vi "Fetch Multi Eval Meas List Segment Total TX Power Results.vi"(6 "Segment (1)":T2=1, 8 "error in (no error)":errorcluster, 9 "Result Type (Current)":i32(ring) items=["Current"=0, "Average"=1, "Standard Deviation"=3, "Maximum"=4, "Minimum"=5], 10 "Instance (1)":T3=1, 11 "VISA resource name":refnum<visa-resource-name>) -> (0 "error out":errorcluster, 1 "TX Power":dbl format="%^.3e", 2 "Reliability":T1, 3 "VISA resource name out":refnum<visa-resource-name>, 4 "Expired Statistics":i32, 5 "Out Of Tolerance":i32)   [LabVIEW 2020, in "Rohde&Schwarz CMWXP NR FR1 Measurement.lvlib"]
doc: "Return total TX power results for segment <no> in list mode.\n\nAttributes:\nRSCMWXPNRFR1M_ATTR_FETCH_MULTI_EVAL_MEAS_LIST_SEGMENT_TOTAL_TX_POWER_CURRENT_RESULTS\nRSCMWXPNRFR1M_ATTR_FETCH_MULTI_EVAL_MEAS_LIST_SEGMENT_TOTAL_TX_POWER_AVERAGE_RESULTS\nRSCMWXPNRFR1M_ATTR_FETCH_MULTI_EVAL_MEAS_LIST_SEGMENT_TOTAL_TX_POWER_STANDARD_DEVIATION_RESULTS\nRSCMWXPNRFR1M_ATTR_FETCH_MULTI_EVAL_MEAS_LIST_SEGMENT_TOTAL_TX_POWER_MAXIMUM_RESULTS\nRSCMWXPNRFR1M_ATTR_FETCH_MULTI_EVAL_MEAS_LIST_SEGMENT_TOTAL_TX_POWER_MINIMUM_RESULTS\n\nRemote-control commands:\nFETCh:NRSub:MEAS<i>:MEValuation:LIST:SEGMent<no>:POWer:CURRent?\nFETCh:NRSub:MEAS<i>:MEValuation:LIST:SEGMent<no>:POWer:AVERage?\nFETCh:NRSub:MEAS<i>:MEValuation:LIST:SEGMent<no>:POWer:SDEViation?\nFETCh:NRSub:MEAS<i>:MEValuation:LIST:SEGMent<no>:POWer:MAXimum?\nFETCh:NRSub:MEAS<i>:MEValuation:LIST:SEGMent<no>:POWer:MINimum?"
uses:
  <instrlib>/Rohde&Schwarz CMWXP NR FR1 Measurement/Rohde&Schwarz CMWXP NR FR1 Measurement.lvlib
  <instrlib>/Rohde&Schwarz CMWXP NR FR1 Measurement/Private/_Instance.ctl
  <instrlib>/Rohde&Schwarz CMWXP NR FR1 Measurement/Private/_Segment.ctl
  <instrlib>/Rohde&Schwarz CMWXP NR FR1 Measurement/Private/_SegReliability.ctl
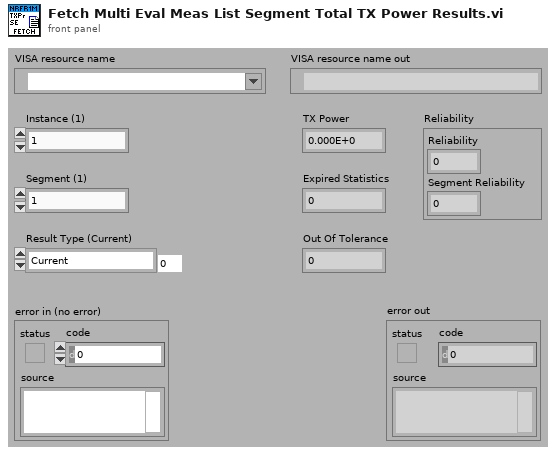
[diagram p1: front panel]
types:
  T1 = typedef "Rohde&Schwarz CMWXP NR FR1 Measurement.lvlib/_SegReliability.ctl" = cluster{"Reliability":i32, "Segment Reliability":i32}
  T2 = typedef "Rohde&Schwarz CMWXP NR FR1 Measurement.lvlib/_Segment.ctl" = i32
  T3 = typedef "Rohde&Schwarz CMWXP NR FR1 Measurement.lvlib/_Instance.ctl" = i32
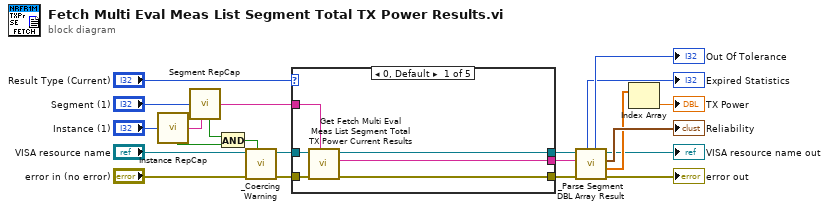
[diagram p0: block diagram]
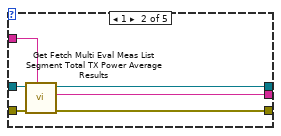
[diagram p2: hidden frame]
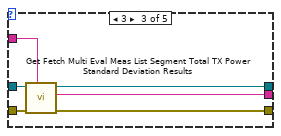
[diagram p3: hidden frame]
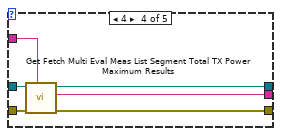
[diagram p4: hidden frame]
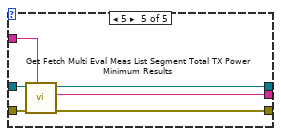
[diagram p5: hidden frame]
diagram:
  n1 = call <instrlib>:"Instance RepCap.vi"("Instance In"="Instance (1)") -> ("In Range?"=w17:bool, "RepCap Identifier Out"=w16:string)  [unwired: 1 in]
  n2 = call <instrlib>:"Segment RepCap.vi"("Segment In"="Segment (1)", "RepCap String In (\"\")"=w16) -> ("In Range?"=w15:bool, "RepCap Identifier Out"=w14:string)
  n3 = And(x=w15, y=w17) -> (x .and. y?=w18:bool)
  n4 = call <instrlib>:"_Coercing Warning.vi"("In Range?"=w18, "error in (no error)"="error in (no error)", "VISA resource name"="VISA resource name") -> ("error out"=w12:errorcluster, "VISA resource name out"=w13:refnum<visa-resource-name>)  [unwired: 7 in]
  n5 = case shown="0, Default" "Result Type (Current)" {
    tunnel: w14 -> [w28 w34 w40 w46 w52]
    tunnel: w13 -> [w27 w33 w39 w45 w51]
    tunnel: w12 -> [w26 w32 w38 w44 w50]
    tunnel: [w25 w31 w37 w43 w49] -> w11
    tunnel: [w24 w30 w36 w42 w48] -> w10
    tunnel: [w23 w29 w35 w41 w47] -> w9
    frame 0, Default {
      n6 = call "Get Fetch Multi Eval Meas List Segment Total TX Power Current Results"("Repeated Capabilities"=w28, "error in (no error)"=w26, "instrument handle"=w27) -> ("error out"=w23:errorcluster, "Fetch Multi Eval Meas List Segment Total TX Power Current Results"=w24:string, "instrument handle out"=w25:refnum<visa-resource-name>)  [unwired: 6 in]
    }
    frame 1 {
      n7 = call "Get Fetch Multi Eval Meas List Segment Total TX Power Average Results"("Repeated Capabilities"=w34, "error in (no error)"=w32, "instrument handle"=w33) -> ("error out"=w29:errorcluster, "Fetch Multi Eval Meas List Segment Total TX Power Average Results"=w30:string, "instrument handle out"=w31:refnum<visa-resource-name>)  [unwired: 6 in]
    }
    frame 3 {
      n8 = call "Get Fetch Multi Eval Meas List Segment Total TX Power Standard Deviation Results"("Repeated Capabilities"=w40, "error in (no error)"=w38, "instrument handle"=w39) -> ("error out"=w35:errorcluster, "Fetch Multi Eval Meas List Segment Total TX Power Standard Deviation Results"=w36:string, "instrument handle out"=w37:refnum<visa-resource-name>)  [unwired: 6 in]
    }
    frame 4 {
      n9 = call "Get Fetch Multi Eval Meas List Segment Total TX Power Maximum Results"("Repeated Capabilities"=w46, "error in (no error)"=w44, "instrument handle"=w45) -> ("error out"=w41:errorcluster, "Fetch Multi Eval Meas List Segment Total TX Power Maximum Results"=w42:string, "instrument handle out"=w43:refnum<visa-resource-name>)  [unwired: 6 in]
    }
    frame 5 {
      n10 = call "Get Fetch Multi Eval Meas List Segment Total TX Power Minimum Results"("Repeated Capabilities"=w52, "error in (no error)"=w50, "instrument handle"=w51) -> ("error out"=w47:errorcluster, "Fetch Multi Eval Meas List Segment Total TX Power Minimum Results"=w48:string, "instrument handle out"=w49:refnum<visa-resource-name>)  [unwired: 6 in]
    }
  }
  n11 = call <instrlib>:"_Parse Segment DBL Array Result.vi"("error in (no error)"=w9, "Input String"=w10, "VISA resource name"=w11) -> ("error out"=→"error out":errorcluster, "Results"=w7:dbl[], "Reliability Results"=→"Reliability":T1, "VISA resource name out"=→"VISA resource name out":refnum<visa-resource-name>, "Out Of Tolerance"=→"Out Of Tolerance":i32, "Statistic Expired"=→"Expired Statistics":i32)  [unwired: 3 in]
  n12 = Index Array(array=w7) -> (element=→"TX Power":dbl)  [unwired: 1 in]
